vi "test_daq_caller.vi"() -> ()   [LabVIEW 2018]
panel:
  in  "Requests":string[](array[string])
  out "error out":errorcluster
  out "outputs":string[](array[string])
  in  "error in":errorcluster
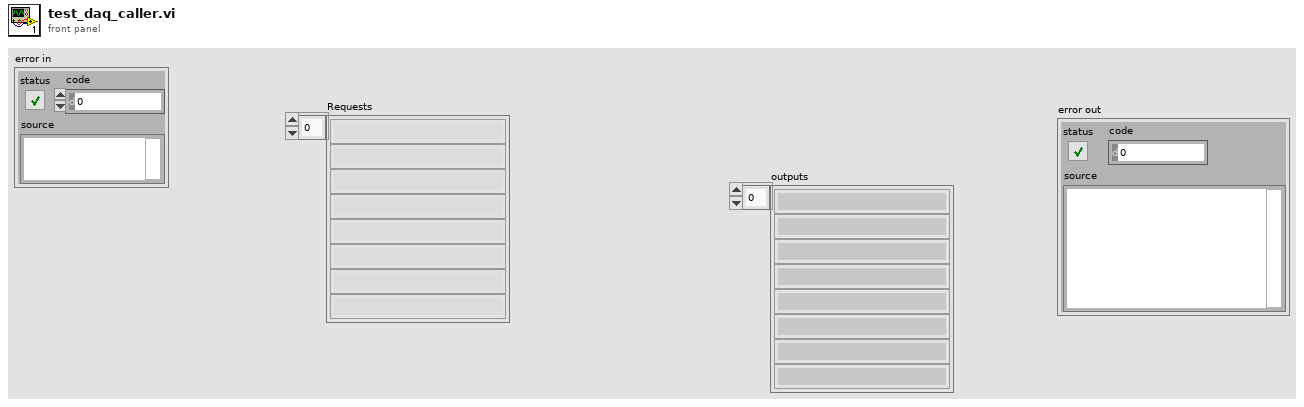
[diagram p1: front panel]
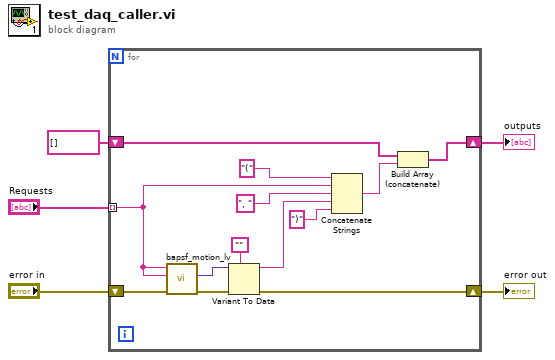
[diagram p0: block diagram]
diagram:
  n1 = for {
    tunnel: "Requests" -> [w13] mode=indexing
    shift-right: [w6] -> w3
    shift-left: "error in" -> [w18]
    shift-right: [w8] -> w4
    shift-left: string[] [] -> [w7]
    n2 = call "bapsf_motion_lv.vi"("error in"=w18, "Request data"=w13, "Request"=w13) -> ("error out"=w17:errorcluster, "Response data"=w16:variant)  [unwired: 3 in]
    n3 = Variant To Data(error in=w17, type="", Variant=w16) -> (data=w11:string, error out=w6:errorcluster)
    n4 = Concatenate Strings("(" ("string"), w13, ", " ("string"), w11, ")" ("string")) -> (w9:string)
    n5 = Build Array (concatenate)(w7, w9) -> (w8:string[])
  }
  "outputs" <- w4
  "error out" <- w3
